vi "Engine Out - Faults - Generic Fault.vi"(11 "Generic [Unit]":sgl) -> ()   [LabVIEW 2015, in "ECS-RT.lvlib"]
uses:
  ECS-RT.lvlib
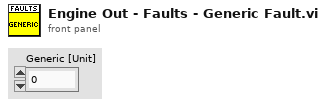
[diagram p1: front panel]
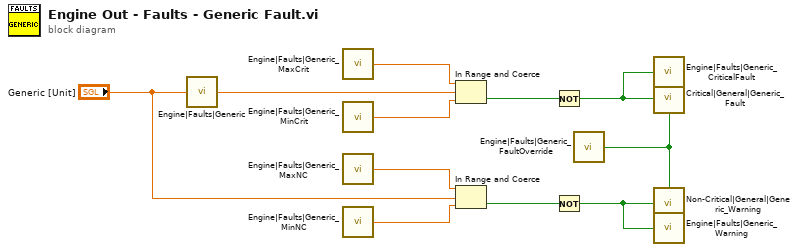
[diagram p0: block diagram]
diagram:
  n1 = call "Engine|Faults|Generic"("Value"="Generic [Unit]") -> ()
  n2 = call "Engine|Faults|Generic_MaxCrit"() -> ("Value"=w3:sgl)
  n3 = call "Engine|Faults|Generic_MinCrit"() -> ("Value"=w4:sgl)
  n4 = call "Engine|Faults|Generic_MaxNC"() -> ("Value"=w7:sgl)
  n5 = call "Engine|Faults|Generic_MinNC"() -> ("Value"=w8:sgl)
  n6 = In Range and Coerce(upper limit=w3, x="Generic [Unit]", lower limit=w4) -> (In Range?=w5:bool)  [unwired: 1 out]
  n7 = In Range and Coerce(upper limit=w7, x="Generic [Unit]", lower limit=w8) -> (In Range?=w9:bool)  [unwired: 1 out]
  n8 = Not(x=w5) -> (.not. x?=w6:bool)
  n9 = Not(x=w9) -> (.not. x?=w10:bool)
  n10 = call "Engine|Faults|Generic_FaultOverride"() -> ("Value"=w1:bool)
  n11 = call "Engine|Faults|Generic_CriticalFault"("Value"=w6) -> ()
  n12 = call "Critical|General|Generic_Fault"("Fault"=w6, "Override (F)"=w1) -> ()  [unwired: 1 in]
  n13 = call "Non-Critical|General|Generic_Warning"("Fault"=w10, "Override (F)"=w1) -> ()  [unwired: 1 in]
  n14 = call "Engine|Faults|Generic_Warning"("Value"=w10) -> ()
